vi "Climber Controller.vi"(8 "error in":errorcluster) -> ()   [LabVIEW 2017]
doc: "This VI executes continuously carrying out the current operation and responding to updates or new operations. It will often contain the timing or control code that is difficult to place directly in TeleOp. This VI generally opens all sensors and motors and isolates the rest of the robot code from knowing how the operations are carried out."
uses:
  <vilib>/Rock Robotics/WPI/Framework/Completion Status.ctl
  Climber Setpoints.ctl
  Climber Operations.ctl
  Public/Documents/Cross The Road Electronics/Phoenix-LabVIEW/Motor Controller/Controls/CTRE_Phoenix_MotorControl_ControlMode.ctl
  Public/Documents/Cross The Road Electronics/Phoenix-LabVIEW/Motor Controller/Controls/CTRE_Phoenix_MotorControl_NeutralMode.ctl
  <vilib>/Rock Robotics/Network Tables/NT Write Boolean.vi
panel:
  in  "Interactive Values":T1
  out "Current\nCmd":string
  in  "Buttons":cluster{"Execute Cmd":bool, "Abort Cmd":bool}
  out "Command Timing":cluster{"Start Time (ms)":u32, "Iterations":i32}
  out "Status":T3
  # "Tip: It may be helpful to observe inputs and sensor values.\nYou may also want to display tuning or debugging controls."
  # "Interactive Command: You may fill in the settings for a command\nand schedule it with the Execute button. You can observe and abort\nany command while fine tuning the code for the controller."
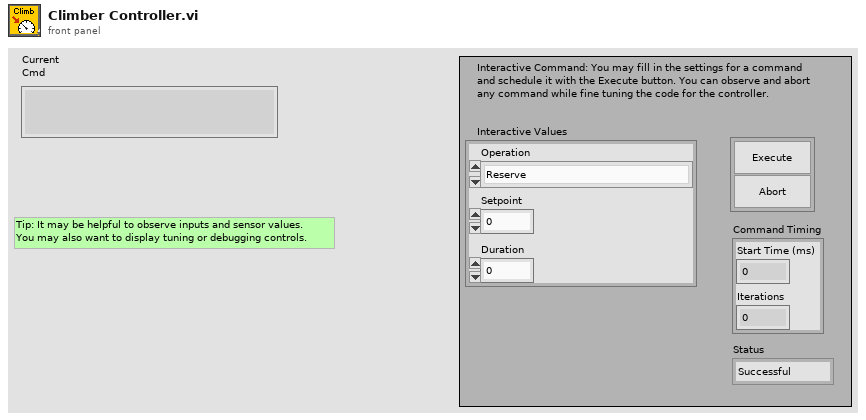
[diagram p1: front panel]
types:
  T1 = typedef "Climber Setpoints.ctl" = cluster{"Operation":T2, "Setpoint":dbl, "Duration":dbl}
  T2 = typedef "Climber Operations.ctl" = enum16{"Reserve", "Read Current", "Immediate", "Climb"}
  T3 = typedef "Completion Status.ctl" = enum16{"Successful", "Aborted", "Incomplete"}
  T4 = typedef "CTRE_Phoenix_MotorControl_NeutralMode.ctl" = enum8{"EEPROMSetting", "Override to Coast", "Override to Brake"}
  T5 = typedef "CTRE_Phoenix_MotorControl_ControlMode.ctl" = u16
  T6 = typedef "WPI_MotorControlDeviceRef.ctl" = cluster{"DeviceStatus":errorcluster, "Type":T7, "PWM":cluster{"PWM Channel":T8, "DeadBand":T9}, "CAN":cluster{"Device Number":u8, "SetOutput VI Ref":variant, "GetOutput VI Ref":variant, "Enable VI Ref":variant, "Disable VI Ref":variant, "Data":variant}, "Invert":bool, "DIO PWM":cluster{"PWM \"Enable\" Channel":T8, "DIOChannel":T10, "PWM Rate":dbl}}
  T7 = typedef "WPI_MotorControlType.ctl" = enum16{"PWM", "CAN", "DIO PWM"}
  T8 = typedef "FPGA_DIOPWMChannel.ctl" = enum8{"PWM 0", "PWM 1", "PWM 2", "PWM 3", "PWM 4", "PWM 5", "PWM 6", "PWM 7", "PWM 8", "PWM 9", "PWM MXP 0", "PWM MXP 1", "PWM MXP 2", "PWM MXP 3", "PWM MXP 4", "PWM MXP 5", "PWM MXP 6", "PWM MXP 7", "PWM MXP 8", "PWM MXP 9", "Invalid"}
  T9 = typedef "WPI_PWMDeadband.ctl" = cluster{"Name":string, "maxPositivePwm":i32, "minPositivePwm":i32, "centerPwm":i32, "maxNegativePwm":i32, "minNegativePwm":i32, "angularRange":u16}
  T10 = typedef "FPGA_DIOChannel.ctl" = enum8{"DIO 0", "DIO 1", "DIO 2", "DIO 3", "DIO 4", "DIO 5", "DIO 6", "DIO 7", "DIO 8", "DIO 9", "DIO MXP 0", "DIO MXP 1", "DIO MXP 2", "DIO MXP 3", "DIO MXP 4", "DIO MXP 5", "DIO MXP 6", "DIO MXP 7", "DIO MXP 8", "DIO MXP 9", "DIO MXP 10", "DIO MXP 11", "DIO MXP 12", "DIO MXP 13", "DIO MXP 14", "DIO MXP 15", "SPI Port CS1", "SPI Port CS2", "SPI Port CS3", "SPI Port MISO", "SPI Port MOSI", "Invalid"}
  T11 = typedef "Command Status Info.ctl" = cluster{"Name":string, "Status":T3, "notifier out":T12}
  T12 = typedef "Completion Notifier.ctl" = refnum<notifier>
  T13 = cluster{"Current Command":T1, "Command Timing":cluster{"Start Time (ms)":u32, "Iterations":i32}, "Command Arguments":cluster{"Command Info":T11, "Description":string, "Default Command":T1, "queue out":refnum<queue>, "Subsystem Name":string}}
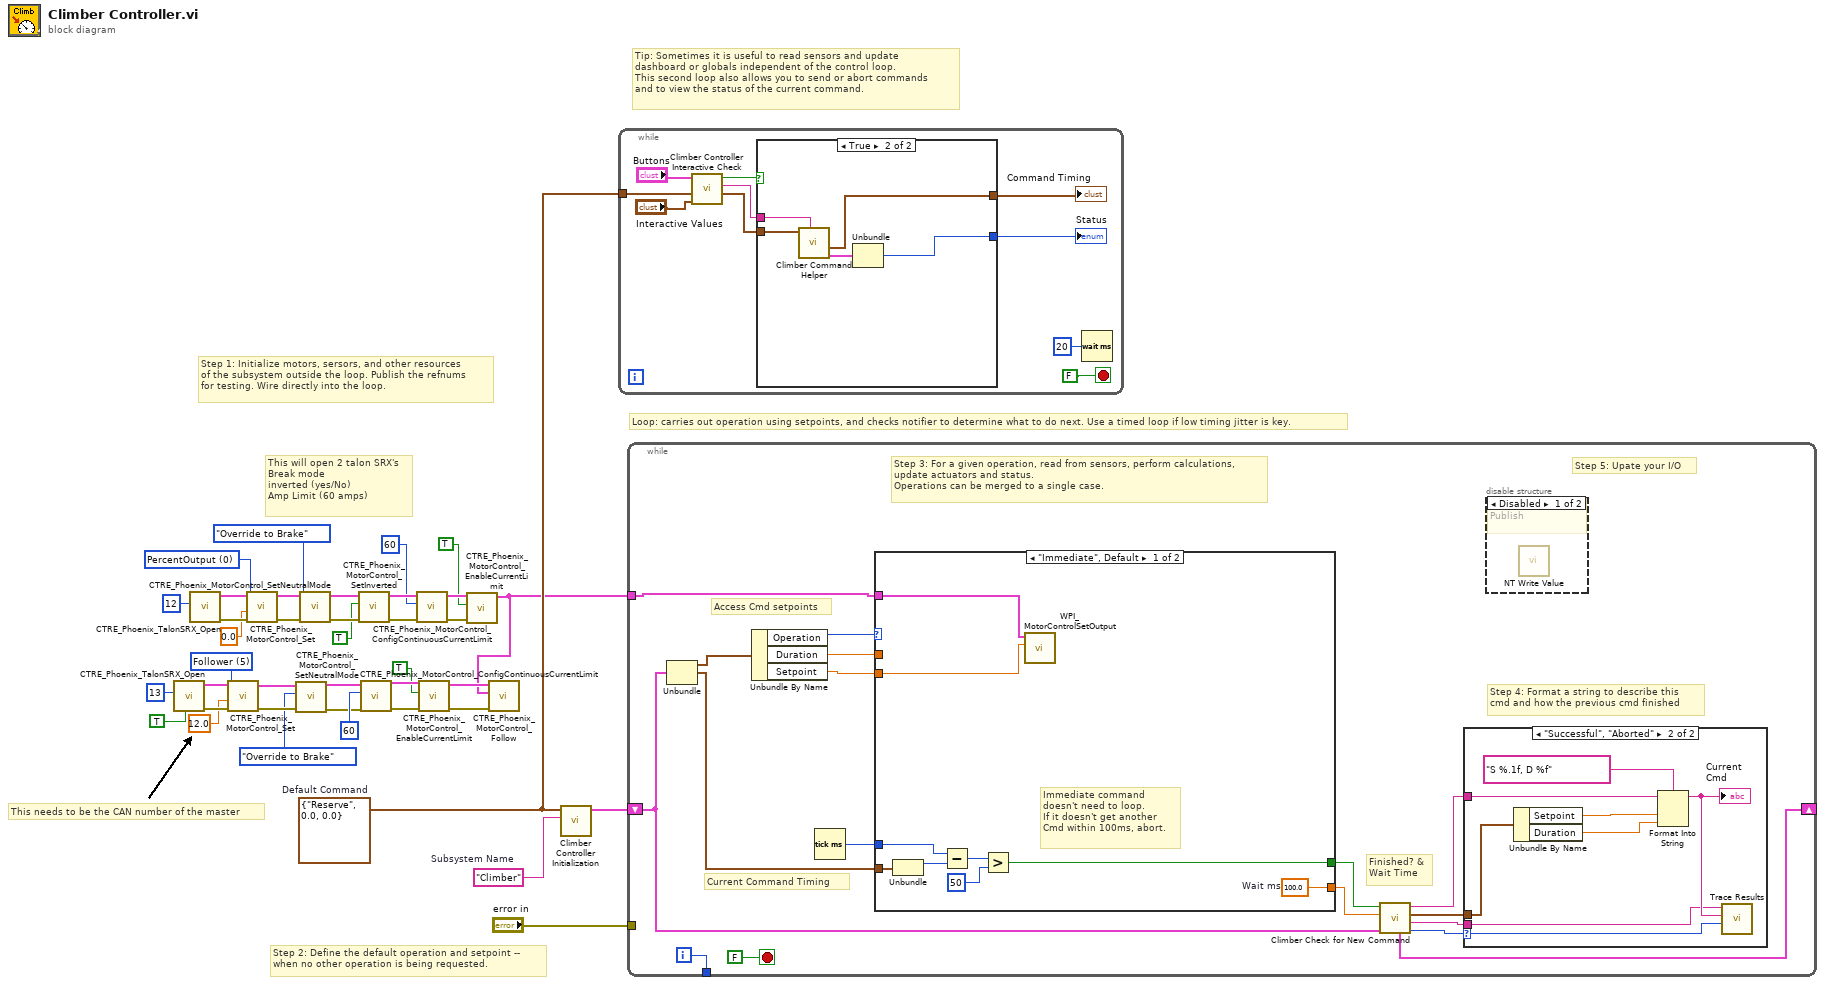
[diagram p0: block diagram]
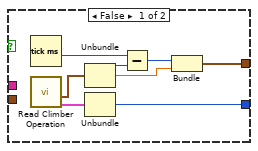
[diagram p2: hidden frame]
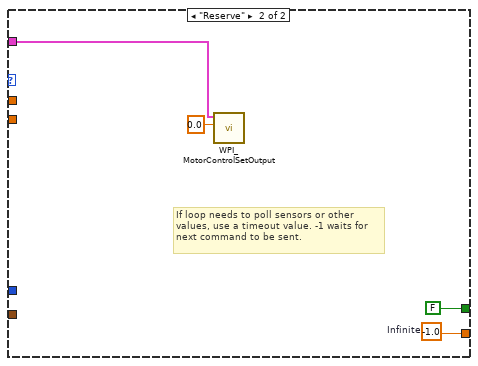
[diagram p5: hidden frame]
diagram:
  w21 = T5 5 items=["PercentOutput"=0, "Position"=1, "Velocity"=2, "Follower"=5, "MotionProfile"=6, "MotionMagic"=7, "MotionMagicArc"=8, "TimedPercentOutput"=9, "Disabled"=15] ("Control Mode")
  w33 = T5 0 items=["PercentOutput"=0, "Position"=1, "Velocity"=2, "Follower"=5, "MotionProfile"=6, "MotionMagic"=7, "MotionMagicArc"=8, "TimedPercentOutput"=9, "Disabled"=15] ("Control Mode")
  w36 = T1 {"Operation"=enum."Reserve", "Setpoint"=0.0, "Duration"=0.0}  # Default Command
  w37 = "Climber"  # Subsystem Name
  # "This needs to be the CAN number of the master"
  # "This will open 2 talon SRX's\nBreak mode\ninverted (yes/No)\nAmp Limit (60 amps)"
  # "Tip: Sometimes it is useful to read sensors and update\ndashboard or globals independent of the control loop.\nThis second loop also allows you to send or abort commands\nand to view the status of the current command."
  # "Step 2: Define the default operation and setpoint --\nwhen no other operation is being requested."
  # "Step 1: Initialize motors, sersors, and other resources\nof the subsystem outside the loop. Publish the refnums\nfor testing. Wire directly into the loop."
  # "Loop: carries out operation using setpoints, and checks notifier to determine what to do next. Use a timed loop if low timing jitter is key."
  n1 = call "CTRE_Phoenix_TalonSRX_Open.vi"("Invert"=TRUE, "Device Number"=u8 13) -> ("error out"=w23:errorcluster, "CAN Talon SRX Ref"=w22:T6)  [unwired: 8 in]
  n2 = call "CTRE_Phoenix_TalonSRX_Open.vi"("Device Number"=u8 12) -> ("error out"=w35:errorcluster, "CAN Talon SRX Ref"=w34:T6)  [unwired: 9 in]
  n3 = call "CTRE_Phoenix_MotorControl_Set.vi"("error in (no error)"=w23, "Output"=12.0, "Control Mode"=w21, "PhoenixMotorControlDevRef"=w22) -> ("error out"=w7:errorcluster, "PhoenixMotorControlDevRef"=w8:T6)  [unwired: 6 in]
  n4 = call "CTRE_Phoenix_MotorControl_Set.vi"("error in (no error)"=w35, "Output"=0.0, "Control Mode"=w33, "PhoenixMotorControlDevRef"=w34) -> ("error out"=w30:errorcluster, "PhoenixMotorControlDevRef"=w29:T6)  [unwired: 6 in]
  n5 = call "CTRE_Phoenix_MotorControl_SetNeutralMode.vi"("error in (no error)"=w7, "Motor Control Neutral Mode"=CTRE_Phoenix_MotorControl_NeutralMode."Override to Brake", "PhoenixMotorControlDevRef"=w8) -> ("error out"=w6:errorcluster, "PhoenixMotorControlDevRef"=w5:T6)  [unwired: 7 in]
  n6 = call "CTRE_Phoenix_MotorControl_SetNeutralMode.vi"("error in (no error)"=w30, "Motor Control Neutral Mode"=CTRE_Phoenix_MotorControl_NeutralMode."Override to Brake", "PhoenixMotorControlDevRef"=w29) -> ("error out"=w27:errorcluster, "PhoenixMotorControlDevRef"=w26:T6)  [unwired: 7 in]
  n7 = call "CTRE_Phoenix_MotorControl_SetInverted.vi"("error in (no error)"=w27, "Invert?"=TRUE, "PhoenixMotorControlDevRef"=w26) -> ("error out"=w2:errorcluster, "PhoenixMotorControlDevRef"=w18:T6)  [unwired: 7 in]
  n8 = call "CTRE_Phoenix_MotorControl_ConfigContinuousCurrentLimit.vi"("error in (no error)"=w6, "Continuous Current Limit (Amps)"=60, "PhoenixMotorControlDevRef"=w5) -> ("error out"=w13:errorcluster, "PhoenixMotorControlDevRef"=w12:T6)  [unwired: 7 in]
  n9 = call "CTRE_Phoenix_MotorControl_ConfigContinuousCurrentLimit.vi"("error in (no error)"=w2, "Continuous Current Limit (Amps)"=60, "PhoenixMotorControlDevRef"=w18) -> ("error out"=w1:errorcluster, "PhoenixMotorControlDevRef"=w15:T6)  [unwired: 7 in]
  n10 = call "CTRE_Phoenix_MotorControl_EnableCurrentLimit.vi"("error in (no error)"=w13, "Enable Current Limit?"=TRUE, "PhoenixMotorControlDevRef"=w12) -> ("error out"=w10:errorcluster, "PhoenixMotorControlDevRef"=w11:T6)  [unwired: 7 in]
  n11 = call "CTRE_Phoenix_MotorControl_EnableCurrentLimit.vi"("error in (no error)"=w1, "Enable Current Limit?"=TRUE, "PhoenixMotorControlDevRef"=w15) -> ("PhoenixMotorControlDevRef"=w3:T6)  [unwired: 7 in, 1 out]
  n12 = call "CTRE_Phoenix_MotorControl_Follow.vi"("error in (no error)"=w10, "Master Controller to Follow"=w3, "PhoenixMotorControlDevRef"=w11) -> ()  [unwired: 7 in, 2 out]
  n13 = call "Climber Controller Initialization.vi"("Subsystem Name"=w37, "Default Command"=w36) -> ("Current Command"=w38:T13)  [unwired: 9 in]
  n14 = while {
    tunnel: w36 -> [w46]
    stop <- FALSE stop-if-true
    n15 = call "Climber Controller Interactive Check.vi"("Interactive Command in"="Interactive Values", "Default Command"=w46, "Buttons"="Buttons") -> ("Interactive Command out"=w43:T1, "Trace String"=w44:string, "Schedule"=w45:bool)  [unwired: 6 in]
    n16 = case shown="True" w45 {
      tunnel: [w57 w62] -> w42
      tunnel: w43 -> [_ w60]
      tunnel: [w53 w58] -> w41
      tunnel: w44 -> [_ w61]
      frame False {
        n17 = Tick Count (ms)() -> (millisecond timer value=w52:u32)
        n18 = call "Read Climber Operation.vi"() -> ("Command Info"=w50:T11, "SubSystem Data"=w51:T1)  [unwired: 9 in, 1 out]
        n19 = Unbundle(w51) -> ("Operation"=w56:T2, "Setpoint"=w54:dbl)  [unwired: 1 out]
        n20 = Unbundle(w50) -> ("Status"=w57:T3)  [unwired: 2 out]
        n21 = Subtract(x=w52, y=w56) -> (x-y=w55:u32)
        n22 = Bundle(w55, "Setpoint"=w54) -> (w53:cluster{u32, "Setpoint":dbl})  [unwired: 1 in]
      }
      frame True {
        n23 = call "Climber Command Helper.vi"("Description"=w61, "SubSystem Data"=w60) -> ("Command Info Out"=w59:T11, "Command Timing"=w58:cluster{"Start Time (ms)":u32, "Iterations":i32})  [unwired: 7 in, 1 out]
        n24 = Unbundle(w59) -> ("Status"=w62:T3)  [unwired: 2 out]
      }
    }
    "Status" <- w42
    "Command Timing" <- w41
    n25 = Wait (ms)(milliseconds to wait=u32 20) -> ()  [unwired: 1 out]
  }
  n26 = while {
    shift-right: [w71] -> _
    shift-left: w38 -> [w64]
    tunnel: [w78] -> _
    tunnel: "error in" -> [_]
    tunnel: w3 -> [w63]
    i -> [w78]
    stop <- FALSE stop-if-true
    # "Step 5: Upate your I/O"
    # "Step 4: Format a string to describe this\ncmd and how the previous cmd finished"
    # "Current Command Timing"
    # "Access Cmd setpoints"
    # "Finished? &\nWait Time"
    # "Step 3: For a given operation, read from sensors, perform calculations,\nupdate actuators and status.\nOperations can be merged to a single case."
    n27 = Unbundle(w64) -> ("Current Command"=w77:T1, "Command Timing"=w73:cluster{"Start Time (ms)":u32, "Iterations":i32})  [unwired: 1 out]
    n28 = Unbundle By Name(w77) -> ("Operation"=w76:T2, "Duration"=w75:dbl, "Setpoint"=w72:dbl)
    n29 = Tick Count (ms)() -> (millisecond timer value=w74:u32)
    n30 = case shown="\"Immediate\", Default" w76 {
      tunnel: [w96 w100] -> w69
      tunnel: [w90 FALSE ("ignore previous (F)")] -> w70
      tunnel: w73 -> [w92 _]
      tunnel: w75 -> [_ _]
      tunnel: w74 -> [w91 _]
      tunnel: w72 -> [w88 _]
      tunnel: w63 -> [w89 w98]
      frame "Immediate", Default {
        w96 = 100.0  # Wait ms
        # "Immediate command\ndoesn't need to loop.\nIf it doesn't get another\nCmd within 100ms, abort."
        n31 = Unbundle(w92) -> ("Start Time (ms)"=w95:u32)  [unwired: 1 out]
        n32 = Subtract(x=w91, y=w95) -> (x-y=w94:u32)
        n33 = Greater?(x=w94, y=u8 50 ("Left Motor")) -> (0:w90:bool)
        n34 = call <vilib>:"WPI_MotorControlSetOutput.vi"("Output"=w88, "MotorControlDevRef"=w89) -> ()  [unwired: 7 in, 3 out]
      }
      frame "Reserve" {
        w100 = -1.0  # Infinite
        # "If loop needs to poll sensors or other\nvalues, use a timeout value. -1 waits for\nnext command to be sent."
        n35 = call <vilib>:"WPI_MotorControlSetOutput.vi"("Output"=0.0, "MotorControlDevRef"=w98) -> ()  [unwired: 7 in, 3 out]
      }
    }
    n36 = call "Climber Check for New Command.vi"("Current Command"=w64, "Wait time (ms)"=w69, "Finished?"=w70) -> ("Completion"=w65:T3, "Subsystem Name"=w66:string, "Current Command"=w67:T1, "Initial Trace String"=w68:string, "NextCommand"=w71:T13)  [unwired: 4 in]
    n37 = case shown="\"Successful\", \"Aborted\"" w65 {
      selector: w65 -> [_ w87]
      tunnel: w68 -> [_ w83]
      tunnel: w67 -> [_ w84]
      tunnel: w66 -> [_ w80]
      frame "Incomplete", Default {
        # "Continuing current command"
      }
      frame "Successful", "Aborted" {
        # "Report and setup for next command"
        n38 = Unbundle By Name(w84) -> ("Setpoint"=w86:dbl, "Duration"=w81:dbl)
        n39 = Format Into String(format string="S %.1f, D %f", initial string=w83, w86, w81) -> (resulting string=w82:string)  [unwired: 1 in, 1 out]
        "Current\nCmd" <- w82
        n40 = call <vilib>:"Trace Results.vi"("Status of previous command"=w87, "Description"=w82, "Subsystem"=w80) -> ()  [unwired: 9 in]
      }
    }
    n41 = disable-structure shown="Disabled" {
      frame Disabled {
        # "Publish"
        n42 = call-poly <vilib>:"NT Write Value.vi"() -> ()  [unwired: 11 in, 1 out]
      }
      frame Enabled {
      }
    }
  }
